vi "MercuryITC-VISA-read-write.vi"(8 "error in (no error)":errorcluster, 10 "write buffer":string, 11 "VISA resource name":refnum<visa-resource-name>) -> (0 "error out":errorcluster, 2 "read buffer":string, 3 "VISA resource name out":refnum<visa-resource-name>)   [LabVIEW 2012]
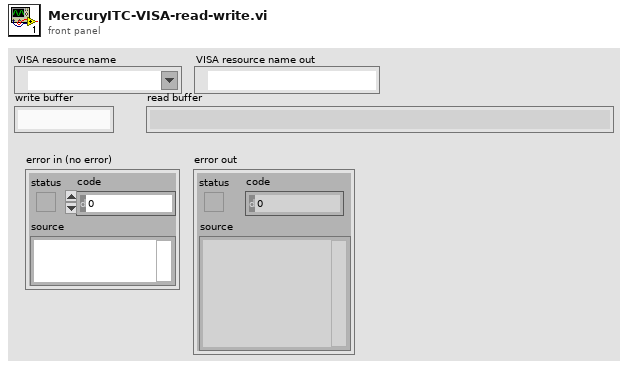
[diagram p1: front panel]
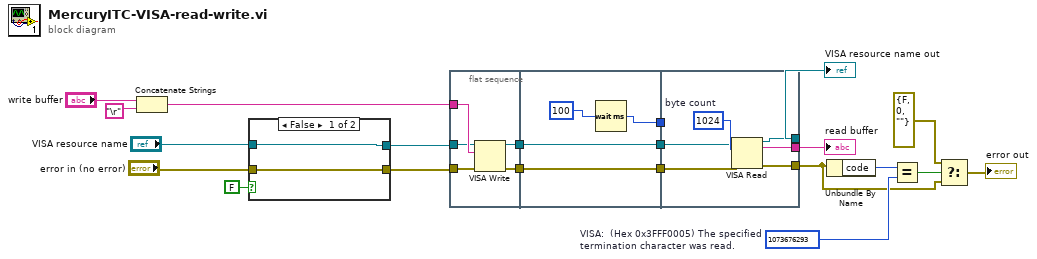
[diagram p0: block diagram]
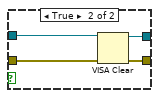
[diagram p2: hidden frame]
diagram:
  w18 = 1073676293  # VISA:  (Hex 0x3FFF0005) The specified termination character was read.
  n1 = Concatenate Strings("write buffer", "\r") -> (w20:string)
  n2 = case shown="False" FALSE {
    tunnel: "VISA resource name" -> [w23 w27]
    tunnel: [w23 w26] -> w5
    tunnel: [w22 w25] -> w4
    tunnel: "error in (no error)" -> [w22 w24]
    frame False {
    }
    frame True {
      n3 = VISA Clear(VISA resource name=w27, error in (no error)=w24) -> (VISA resource name out=w26:refnum<visa-resource-name>, error out=w25:errorcluster)
    }
  }
  n4 = flat-sequence {
    tunnel: w20 -> [w30]
    tunnel: w4 -> [w29]
    tunnel: w5 -> [w28]
    tunnel: [w32] -> w14
    tunnel: [w31] -> w13
    tunnel: w14 -> [w36]
    tunnel: w13 -> [w35]
    tunnel: [w36] -> w12
    tunnel: [w35] -> w11
    tunnel: [w33] -> w2
    tunnel: w12 -> [w40]
    tunnel: w11 -> [w41]
    tunnel: [w39] -> w7
    tunnel: [w38] -> w9
    tunnel: [w37] -> w8
    tunnel: w2 -> [_]
    frame #0 {
      n5 = VISA Write(VISA resource name=w28, write buffer=w30, error in (no error)=w29) -> (VISA resource name out=w31:refnum<visa-resource-name>, error out=w32:errorcluster)  [unwired: 1 out]
    }
    frame #1 {
      n6 = Wait (ms)(milliseconds to wait=u32 100) -> (millisecond timer value=w33:u32)
    }
    frame #2 {
      w42 = u32 1024  # byte count
      n7 = VISA Read(VISA resource name=w41, byte count=w42, error in (no error)=w40) -> (VISA resource name out=w37:refnum<visa-resource-name>, read buffer=w38:string, error out=w39:errorcluster)  [unwired: 1 out]
    }
  }
  n8 = Unbundle By Name(w7) -> ("code"=w10:i32)
  n9 = Equal?(x=w10, y=w18) -> (x = y?=w16:bool)
  n10 = Select(t=errorcluster {"status"=FALSE, "code"=0, "source"=""}, s=w16, f=w7) -> (s? t:f=→"error out":errorcluster)
  "VISA resource name out" <- w8
  "read buffer" <- w9
